vi "ELVIS III v1.0 AO Block Write.vi"(5 "Wait Until Done?":bool, 6 "AO FIFO Sample Rate":dbl=1000.0 min=1000.0 max=1600000.0, 8 "error in (no error)":errorcluster, 9 "dbl Scaled Value List":dbl[][](array[numeric]), 10 "AO (N Samples) Channel List":T3, 11 "myRIO Ref In":T1) -> (0 "error out":errorcluster, 3 "myRIO Ref Out":T1)   [LabVIEW 2021]
uses:
  <vilib>/myRIO/Common/Instrument Driver Framework/myRIO v1.0/AO Block/typedefs/AO Block Channels List.ctl
  <vilib>/myRIO/Common/Instrument Driver Framework/myRIO v1.0/AO Block/typedefs/AO Block Channels Enum.ctl
  <vilib>/myRIO/Common/Instrument Driver Framework/Utilities/typedefs/myRIO v1.0 Reference.ctl
  <vilib>/myRIO/Common/Instrument Driver Framework/Utilities/typedefs/Generic FPGA Reference.ctl
  <vilib>/myRIO/Common/Instrument Driver Framework/ELVIS III v1.0/AO Block/typedefs/ELVIS III AO Block Channels FPGA Reference.ctl
  <vilib>/myRIO/Common/Instrument Driver Framework/ELVIS III v1.0/AO Block/typedefs/ELVIS III AO Block Configuration.ctl
  <vilib>/myRIO/Common/Instrument Driver Framework/ELVIS III v1.0/AO Block/typedefs/ELVIS III AO Block Bank Data.ctl
  <vilib>/myRIO/Common/Instrument Driver Framework/myRIO v1.0/Resource Manager/vis/myRIO v1.0 Block Write Configuration.vi
  <vilib>/rvi/errors/niLvFpgaAdjustHostInterfaceError.vi
  <vilib>/rvi/interface/nirviReadWriteControl/nirviReadWriteControl.xnode
  NiFpgaLv.dll
  <vilib>/rvi/interface/Simulation/niFpgaSimulationCallBeginRW.vi
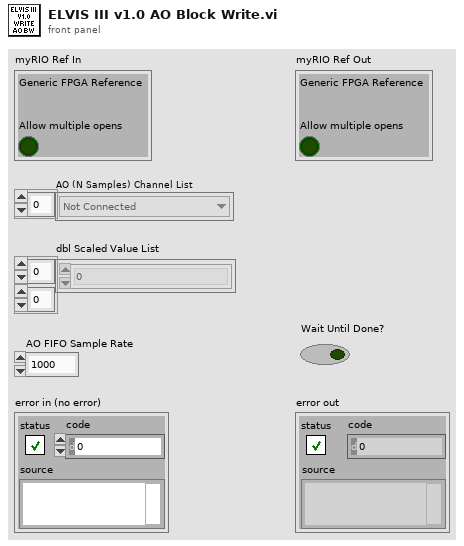
[diagram p1: front panel]
types:
  T1 = typedef "myRIO v1.0 Reference.ctl" = cluster{"Generic FPGA Reference":T2, "Allow multiple opens":bool}
  T2 = typedef "Generic FPGA Reference.ctl" = refnum<k20>
  T3 = typedef "AO Block Channels List.ctl" = T4[]
  T4 = typedef "AO Block Channels Enum.ctl" = enum16{"Not Connected", "A/AO0 (N Samples)", "A/AO1 (N Samples)", "B/AO0 (N Samples)", "B/AO1 (N Samples)"}
  T5 = typedef "ELVIS III AO Block Configuration.ctl" = cluster{"AO FIFO Clock Divisor":u32, "Wait Until Done?":bool, "Write Mode":u8, "AO (N Samples) Configuration ":T6[]}
  T6 = typedef "ELVIS III AO Block Bank Data.ctl" = cluster{"Analog data reference":refnum<data-value>, "Semaphore":T7, "ENA_MASK":u8}
  T7 = typedef "Semaphore RefNum" = refnum<k1>
  T8 = typedef "ELVIS III AO Block Channels FPGA Reference.ctl" = refnum<k20>
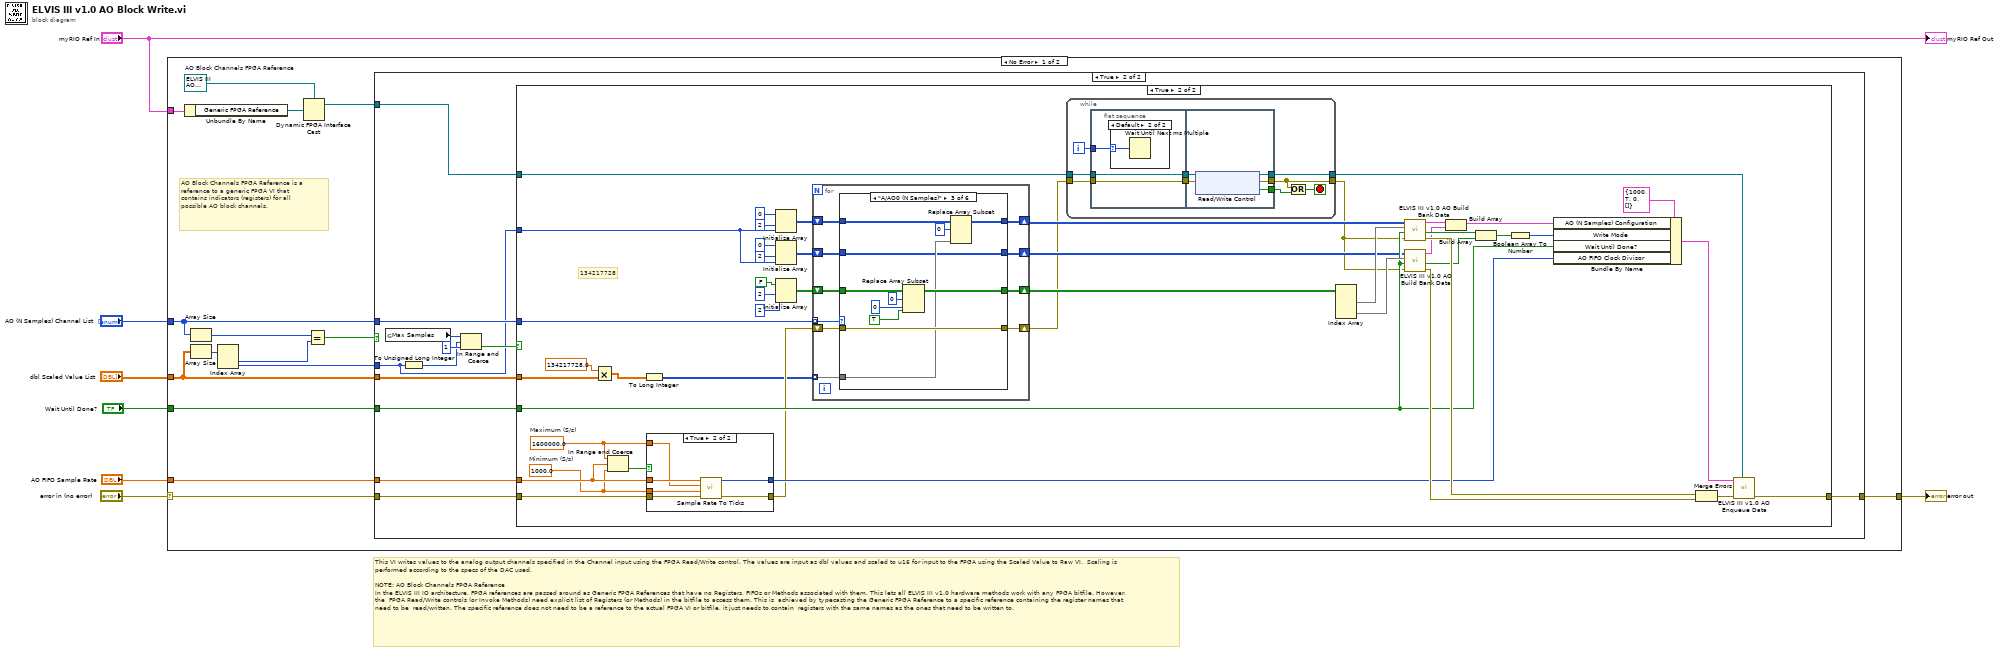
[diagram p0: block diagram]
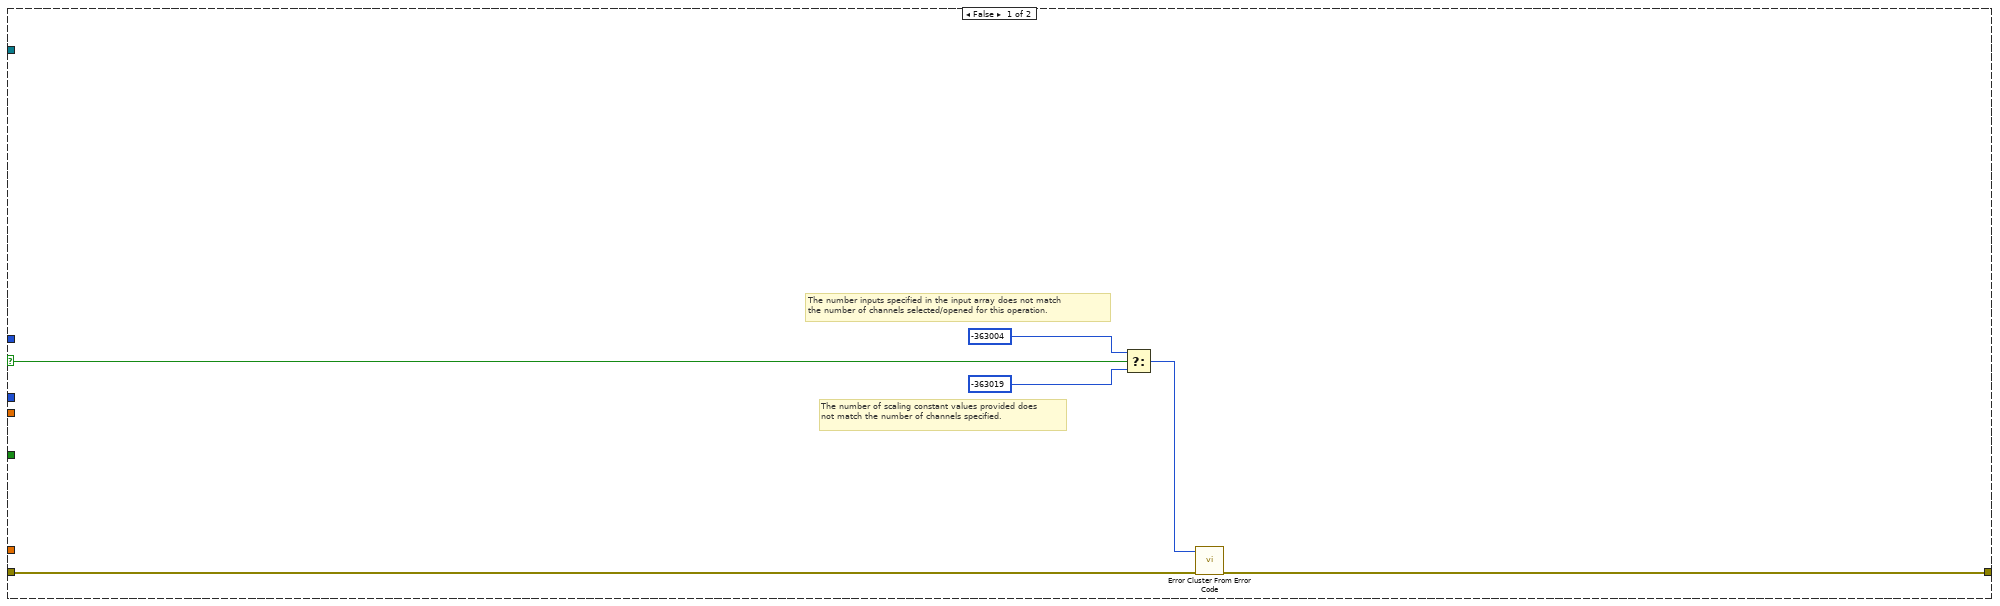
[diagram p2: hidden frame]
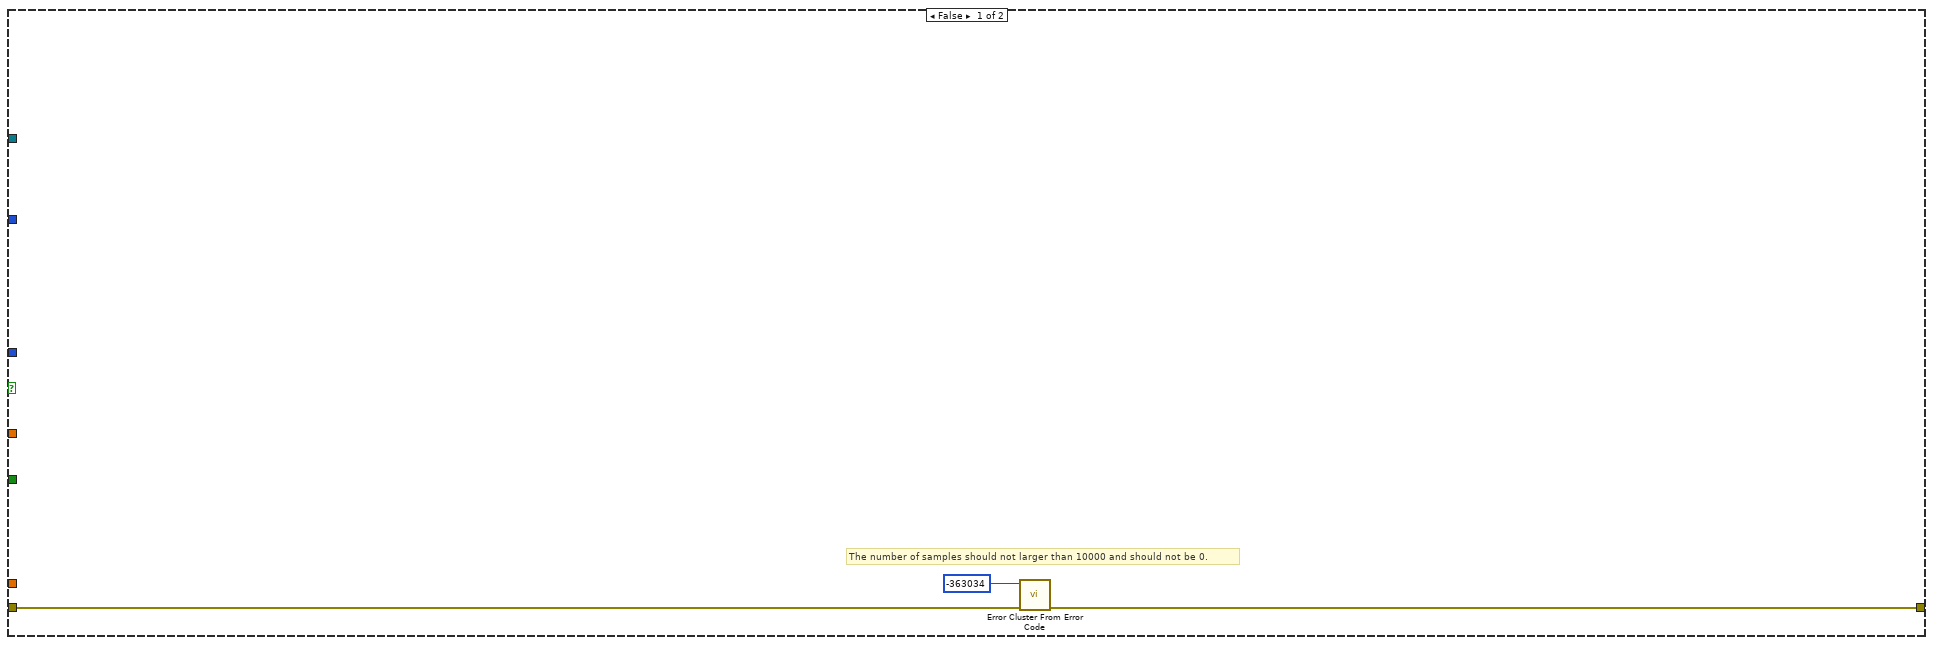
[diagram p3: hidden frame]
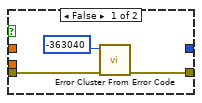
[diagram p5: hidden frame]
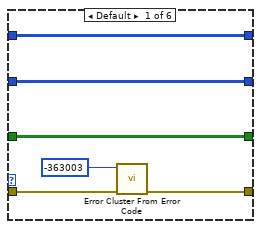
[diagram p6: hidden frame]
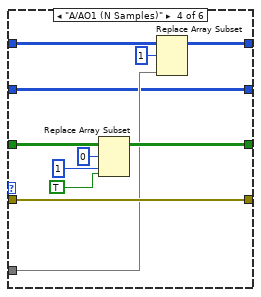
[diagram p8: hidden frame]
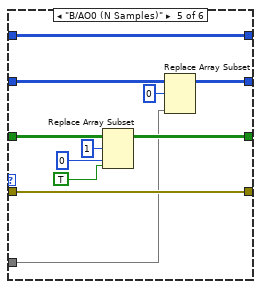
[diagram p9: hidden frame]
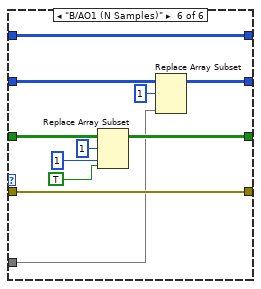
[diagram p10: hidden frame]
diagram:
  # "This VI writes values to the analog output channels specified in the Channel input using the FPGA Read/Write control. The values are input as dbl values and scaled to u16 for input to the FPGA using the Scaled Value to Raw VI.  Scaling is performed according to the specs of the DAC used.\n\nNOTE: AO Block Channels FPGA Reference\nIn the ELVIS III IO architecture, FPGA references are passed around as Generic FPGA References that have no Registers, FIFOs or Methods associated with them. This lets all ELVIS III v1.0 hardware methods work with any FPGA bitfile. However, the  FPGA Read/Write controls (or Invoke Methods) need explicit list of Registers (or Methods) in the bitfile to access them. This is  achieved by typecasting the Generic FPGA Reference to a specific reference containing the register names that need to be  read/written. The specific reference does not need to be a reference to the actual FPGA VI or bitfile, it just needs to contain  registers with the same names as the ones that need to be written to."
  n1 = case shown="No Error" "error in (no error)" {
    selector: "error in (no error)" -> [w8 w181]
    tunnel: [w22 w181] -> w7
    tunnel: "AO (N Samples) Channel List" -> [w21 _]
    tunnel: "dbl Scaled Value List" -> [w20 _]
    tunnel: "AO FIFO Sample Rate" -> [w9 _]
    tunnel: "Wait Until Done?" -> [w17 _]
    tunnel: "myRIO Ref In" -> [w15 _]
    frame No Error {
      w13 = T8 refnum  # AO Block Channels FPGA Reference
      # "AO Block Channels FPGA Reference is a reference to a generic FPGA VI that contains indicators (registers) for all possible AO block channels."
      n2 = Unbundle By Name(w15) -> ("Generic FPGA Reference"=w16:T2)
      n3 = Array Size(array=w21) -> (size(s)=w18:i32)
      n4 = Array Size(array=w20) -> (size(s)=w19:i32[])
      n5 = Index Array(array=w19) -> (element #1=w12:i32, element #2=w11:i32)  [unwired: 2 in]
      n6 = Dynamic FPGA Interface Cast(Session In=w13, Type=w16) -> (Session Out=w14:T8)
      n7 = Equal?(x=w18, y=w12) -> (x = y?=w10:bool)
      n8 = case shown="True" w10 {
        selector: w10 -> [w23 _]
        tunnel: [w28 w39] -> w22
        tunnel: w21 -> [_ w40]
        tunnel: w20 -> [_ w31]
        tunnel: w17 -> [_ w38]
        tunnel: w14 -> [_ w37]
        tunnel: w11 -> [_ w30]
        tunnel: w8 -> [w24 w36]
        tunnel: w9 -> [_ w29]
        frame False {
          # "The number of scaling constant values provided does not match the number of channels specified."
          # "The number inputs specified in the input array does not match\nthe number of channels selected/opened for this operation."
          n9 = Select(t=-363004 ("error code (0)"), s=w23, f=-363019 ("error code (0)")) -> (s? t:f=w25:i32)
          n10 = call <vilib>:"Error Cluster From Error Code.vi"("error in (no error)"=w24, "error code (0)"=w25) -> ("error out"=w28:errorcluster)  [unwired: 7 in]
        }
        frame True {
          n11 = global read "myRIO v1.0 Block Write Configuration.vi" "Max Samples"() -> (w35:u32)
          n12 = To Unsigned Long Integer(number=w30) -> (unsigned 32bit integer=w32:u32)
          n13 = In Range and Coerce(upper limit=w35, x=w32, lower limit=u32 1) -> (In Range?=w33:bool)  [unwired: 1 out]
          n14 = case shown="True" w33 {
            tunnel: w40 -> [_ w84]
            tunnel: [w43 w76] -> w39
            tunnel: w38 -> [_ w59]
            tunnel: w37 -> [_ w50]
            tunnel: w36 -> [w41 w51]
            tunnel: w30 -> [_ w70]
            tunnel: w31 -> [_ w75]
            tunnel: w29 -> [_ w54]
            frame False {
              # "The number of samples should not larger than 10000 and should not be 0."
              n15 = call <vilib>:"Error Cluster From Error Code.vi"("error in (no error)"=w41, "error code (0)"=-363034) -> ("error out"=w43:errorcluster)  [unwired: 7 in]
            }
            frame True {
              w52 = 1000.0  # Minimum (S/s)
              w55 = 1600000.0  # Maximum (S/s)
              # "134217728"
              n16 = Multiply(x=134217728.0, y=w75) -> (x*y=w46:dbl[][])
              n17 = In Range and Coerce(upper limit=w55, x=w54, lower limit=w52) -> (In Range?=w53:bool)  [unwired: 1 out]
              n18 = To Long Integer(number=w46) -> (32bit integer=w44:i32[][])
              n19 = case shown="True" w53 {
                tunnel: [_ w116] -> w57
                tunnel: w51 -> [w109 w115]
                tunnel: [w108 w114] -> w56
                tunnel: w54 -> [_ w113]
                tunnel: w52 -> [_ w112]
                tunnel: w55 -> [_ w111]
                frame False {
                  n20 = call <vilib>:"Error Cluster From Error Code.vi"("error in (no error)"=w109, "error code (0)"=-363040) -> ("error out"=w108:errorcluster)  [unwired: 7 in]
                }
                frame True {
                  n21 = call <vilib>:"Sample Rate To Ticks.vi"("error in (no error)"=w115, "Minimum (S/s)"=w112, "Maximum (S/s)"=w111, "Sample Rate (S/s)"=w113) -> ("error out"=w114:errorcluster, "Count (tick/s)"=w116:u32)  [unwired: 5 in, 1 out]
                }
              }
              n22 = Initialize Array(0, 2 ("dimension size"), w70) -> (w69:i32[][])
              n23 = Initialize Array(0, 2 ("dimension size"), w70) -> (w68:i32[][])
              n24 = Initialize Array(FALSE ("element"), 2 ("dimension size"), 2 ("dimension size")) -> (w86:bool[][])
              n25 = for {
                tunnel: w84 -> [w126] mode=indexing
                shift-right: [w124] -> w85
                shift-left: w86 -> [w125]
                shift-right: [w122] -> w48
                shift-left: w56 -> [w123]
                tunnel: w44 -> [w121] mode=indexing
                shift-right: [w119] -> w65
                shift-left: w69 -> [w120]
                shift-right: [w117] -> w58
                shift-left: w68 -> [w118]
                n26 = case shown="\"A/AO0 (N Samples)\"" w126 {
                  tunnel: w125 -> [w129 w136 w143 w154 w166 w177]
                  tunnel: [w129 w136 w144 w155 w165 w176] -> w124
                  tunnel: w123 -> [w131 w135 w142 w153 w164 w175]
                  tunnel: [w130 w135 w142 w153 w164 w175] -> w122
                  tunnel: w121 -> [_ _ w139 w150 w159 w170]
                  tunnel: w120 -> [w128 w134 w141 w151 w163 w174]
                  tunnel: [w128 w134 w138 w149 w163 w174] -> w119
                  tunnel: w118 -> [w127 w133 w137 w148 w161 w172]
                  tunnel: [w127 w133 w137 w148 w160 w171] -> w117
                  frame Default {
                    n27 = call <vilib>:"Error Cluster From Error Code.vi"("error in (no error)"=w131, "error code (0)"=-363003) -> ("error out"=w130:errorcluster)  [unwired: 7 in]
                  }
                  frame "Not Connected" {
                  }
                  frame "A/AO0 (N Samples)" {
                    n28 = Replace Array Subset(array=w143, new element=TRUE ("new element/subarray"), index (row)=0 ("index"), index (col)=0 ("disabled index (col)")) -> (w144:bool[][])
                    n29 = Replace Array Subset(array=w141, new element=w139, index (row)=0) -> (w138:i32[][])  [unwired: 1 in]
                  }
                  frame "A/AO1 (N Samples)" {
                    n30 = Replace Array Subset(array=w154, new element=TRUE ("new element/subarray"), index (row)=0 ("index"), index (col)=1 ("disabled index (col)")) -> (w155:bool[][])
                    n31 = Replace Array Subset(array=w151, new element=w150, index (row)=1) -> (w149:i32[][])  [unwired: 1 in]
                  }
                  frame "B/AO0 (N Samples)" {
                    n32 = Replace Array Subset(array=w166, new element=TRUE ("new element/subarray"), index (row)=1 ("index"), index (col)=0 ("disabled index (col)")) -> (w165:bool[][])
                    n33 = Replace Array Subset(array=w161, new element=w159, index (row)=0) -> (w160:i32[][])  [unwired: 1 in]
                  }
                  frame "B/AO1 (N Samples)" {
                    n34 = Replace Array Subset(array=w177, new element=TRUE ("new element/subarray"), index (row)=1 ("index"), index (col)=1 ("disabled index (col)")) -> (w176:bool[][])
                    n35 = Replace Array Subset(array=w172, new element=w170, index (row)=1) -> (w171:i32[][])  [unwired: 1 in]
                  }
                }
              }
              n36 = while {
                tunnel: w50 -> [w98]
                tunnel: w48 -> [w97]
                tunnel: [w94] -> w47
                tunnel: [w91] -> w49
                i -> [w90]
                stop <- w92 stop-if-true
                n37 = flat-sequence {
                  tunnel: w97 -> [w100]
                  tunnel: w98 -> [w101]
                  tunnel: [w101] -> w96
                  tunnel: [w100] -> w95
                  tunnel: w90 -> [w99]
                  tunnel: [w105] -> w93
                  tunnel: [w104] -> w94
                  tunnel: w96 -> [w107]
                  tunnel: w95 -> [w106]
                  tunnel: [w103] -> w91
                  frame #0 {
                    n38 = case shown="Default" w99 {
                      selector: w99 -> [_ w102]
                      frame 0 {
                      }
                      frame Default {
                        n39 = Wait Until Next ms Multiple(millisecond multiple=w102) -> ()  [unwired: 1 out]
                      }
                    }
                  }
                  frame #1 {
                    n40 = xnode "Read/Write Control"("FPGA VI Reference In"=w107, "error in"=w106) -> ("FPGA VI Reference Out"=w103:T8, "error out"=w104:errorcluster, "DMA.SYS.RDY"=w105:bool)
                  }
                }
                n41 = Or(x=w94, y=w93) -> (x .or. y?=w92:bool)
              }
              n42 = Index Array(array=w85) -> (element #1=w64:bool[], element #2=w66:bool[])  [unwired: 4 in]
              n43 = call <vilib>:"ELVIS III v1.0 AO Build Bank Data.vi"("error in (no error)"=w47, "Wait Until Done?"=w59, "Channel Bitmask"=w64, "dbl Scaled Value List in"=w65) -> ("error out"=w78:errorcluster, "Channel Selected?"=w62:bool, "Bank Data"=w63:T6)  [unwired: 5 in]
              n44 = call <vilib>:"ELVIS III v1.0 AO Build Bank Data.vi"("error in (no error)"=w47, "Wait Until Done?"=w59, "Channel Bitmask"=w66, "dbl Scaled Value List in"=w58) -> ("error out"=w67:errorcluster, "Channel Selected?"=w60:bool, "Bank Data"=w61:T6)  [unwired: 5 in]
              n45 = Build Array(w63, w61) -> (w80:T6[])
              n46 = Build Array(w62, w60) -> (w83:bool[])
              n47 = Boolean Array To Number(Boolean array=w83) -> (number=w81:u8)
              n48 = Bundle By Name(cluster=T5 {"AO FIFO Clock Divisor"=1000, "Wait Until Done?"=TRUE, "Write Mode"=0, "AO (N Samples) Configuration "=[]} ("ELVIS III AO (N Samples) Configuration"), "AO (N Samples) Configuration"=w80, "Write Mode"=w81, "Wait Until Done?"=w59, "AO FIFO Clock Divisor"=w57) -> (w79:T5)
              n49 = Merge Errors(w78, w67) -> (w77:errorcluster)
              n50 = call <vilib>:"ELVIS III v1.0 AO Enqueue Data.vi"("AO Block Channels FPGA Reference"=w49, "error in (no error)"=w77, "AO Block Write Configuration"=w79) -> ("error out"=w76:errorcluster)  [unwired: 8 in]
            }
          }
        }
      }
    }
    frame Error {
      # "There is an incoming error so there is nothing to do."
    }
  }
  "error out" <- w7
  "myRIO Ref Out" <- "myRIO Ref In"
